vi "ChangeGraphRef.vi"(7 "NewGraphIndex":i32, 8 "error in (no error)":errorcluster caption="entrée d'erreur (pas d'erreur)", 9 "CurveIndex":i32, 11 "Interface en entrée":refnum<class "Interface.lvclass"> caption="DNL_LabVIEW Object in") -> (0 "error out":errorcluster caption="sortie d'erreur", 2 "OldGraphIndex":i32, 3 "Interface en sortie":refnum<class "Interface.lvclass"> caption="DNL_LabVIEW Object out")   [LabVIEW 2010, in "Interface.lvclass"]
uses:
  Interface.lvclass
  Interface.lvclass/Interface.ctl
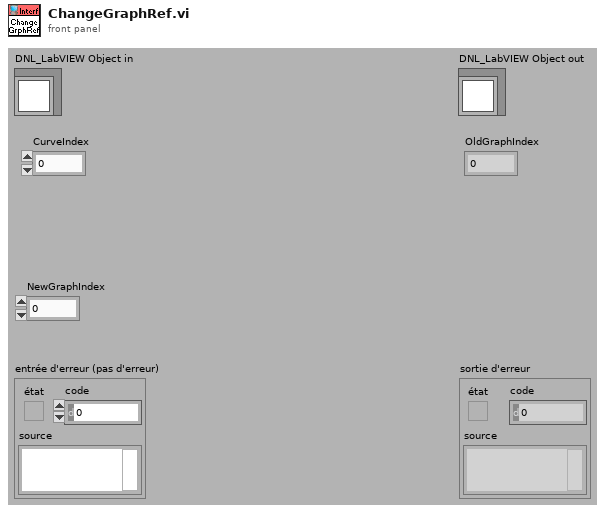
[diagram p1: front panel]
types:
  T1 = typedef "Interface.lvclass/CurveSetup.ctl" = cluster{"CurveName":string, "YParam":string, "XParam":string, "ZParam ":string, "GroupName":string, "LinWdth":u8, "PntCol":u32, "LinCol":u32, "LablFor":u8, "XScale":u32, "YScale":u32, "Interpol":u8, "DisplayName":string, "FillType":i16, "LineStyle":u8, "PntStyle":u8, "BarTyp":u8, "GraphIndex":i32, "Visible":bool, "XScaleName":string, "YScaleName":string, "XYGraph_Ref":refnum<vi>}
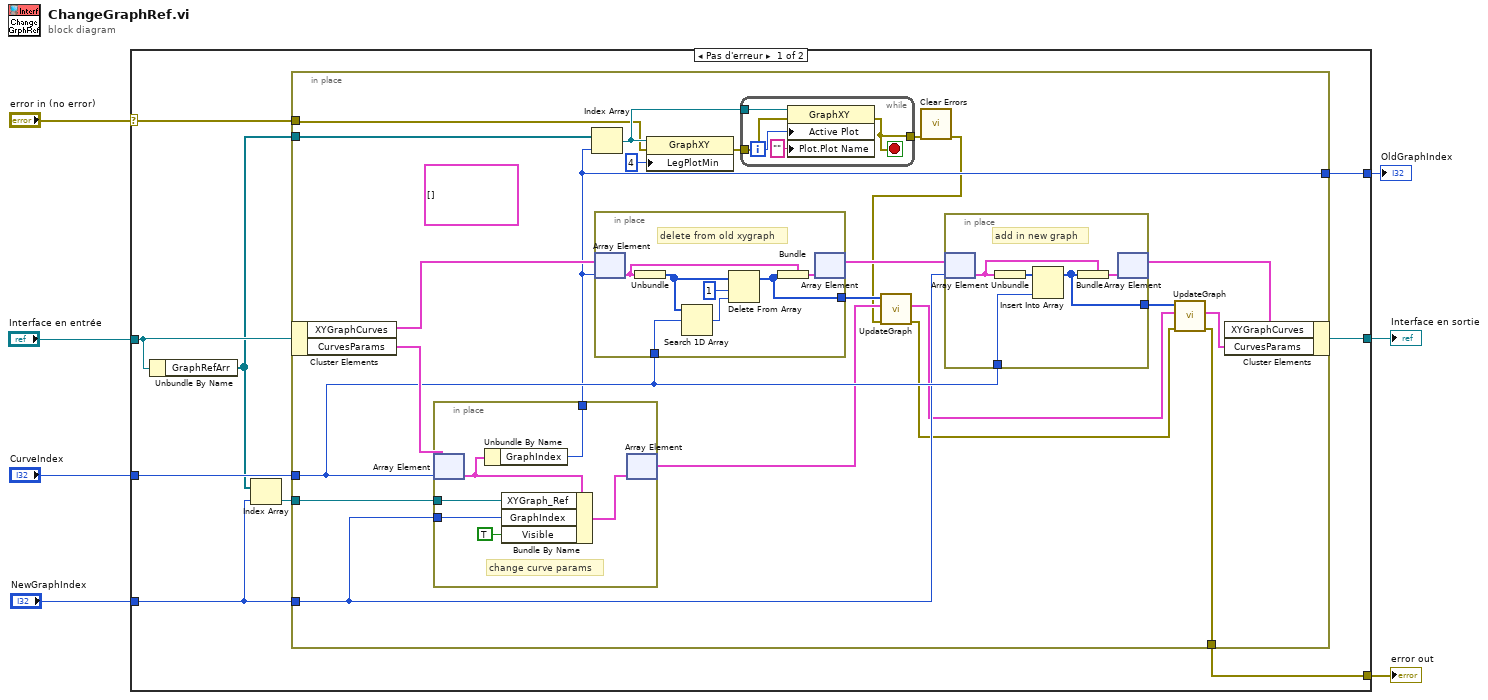
[diagram p0: block diagram]
diagram:
  n1 = case shown="Pas d'erreur" "error in (no error)" {
    selector: "error in (no error)" -> [w15 w63]
    tunnel: [w13 w63] -> w6
    tunnel: [w14 w62] -> w4
    tunnel: "Interface en entrée" -> [w12 w62]
    tunnel: "CurveIndex" -> [w16 _]
    tunnel: "NewGraphIndex" -> [w10 _]
    tunnel: [w9 _] -> w1
    frame No Error {
      n2 = Unbundle By Name(w12) -> ("GraphRefArr"=w8:refnum<vi>[])
      n3 = Index Array(array=w8, index=w10) -> (element=w11:refnum<vi>)
      n4 = in-place {
        in-place-border: w16 -> [w36]
        in-place-border: w11 -> [w37]
        in-place-border: w10 -> [w32]
        in-place-border: w15 -> [w22]
        in-place-border: [w28] -> w13
        in-place-border: [w25] -> w9
        in-place-border: w8 -> [w26]
        (unwired) cluster{dbl[], dbl[]}[] []
        n5 = in-place-cluster #1(w12) -> ("XYGraphCurves"=w35:cluster{"Tableau":i32[]}[], "CurvesParams"=w38:T1[])
        n6 = in-place {
          in-place-border: w37 -> [w60]
          in-place-border: [w58] -> w25
          in-place-border: w32 -> [w57]
          # "change curve params"
          n7 = in-place-array #2(w38, w36) -> (w59:T1)
          n8 = Unbundle By Name(w59) -> ("GraphIndex"=w58:i32)
          n9 = Bundle By Name(cluster=w59, "XYGraph_Ref"=w60, "GraphIndex"=w57, "Visible"=TRUE) -> (w61:T1)
          n10 = in-place-array #2(w61) -> (w29:T1[])  [unwired: 1 out]
        }
        n11 = Index Array(array=w26, index=w25) -> (element=w23:refnum<vi>)
        n12 = in-place {
          in-place-border: w36 -> [w54]
          in-place-border: [w49] -> w31
          # "delete from old xygraph"
          n13 = in-place-array #3(w35, w25) -> (w51:cluster{"Tableau":i32[]})
          n14 = Unbundle(w51) -> ("Tableau"=w52:i32[])
          n15 = Search 1D Array(1D array=w52, element=w54) -> (index of element=w53:i32)  [unwired: 1 in]
          n16 = Delete From Array(array=w52, length=1 ("longueur"), index=w53) -> (array with subset deleted=w49:i32[])  [unwired: 1 out]
          n17 = Bundle(cluster=w51, "Tableau"=w49) -> (w50:cluster{"Tableau":i32[]})
          n18 = in-place-array #3(w50) -> (w34:cluster{"Tableau":i32[]}[])  [unwired: 1 out]
        }
        n19 = property class="GraphXY"(reference=w23, error in=w22, "LegPlotMin"=u32 4 ("Légende : minimum de tracés")) -> (error out=w20:errorcluster)  [unwired: 1 out]
        n20 = while {
          tunnel: w23 -> [w43]
          tunnel: w20 -> [w41]
          tunnel: [w39] -> w19
          i -> [w40]
          stop <- w39 stop-if-true
          n21 = property class="GraphXY"(reference=w43, error in=w41, "Active Plot"=w40, "Plot.Plot Name"="" ("Tracé.Nom du tracé")) -> (error out=w39:errorcluster)  [unwired: 1 out]
        }
        n22 = call <vilib>:"Clear Errors.vi"("error in (no error)"=w19) -> ("error out"=w21:errorcluster)  [unwired: 6 in]
        n23 = call "UpdateGraph.vi"("error in (no error)"=w21, "CurvesParams"=w29, "CurveIndexArr"=w31) -> ("error out"=w27:errorcluster, "CurvesParamsOut"=w18:T1[])  [unwired: 7 in]
        n24 = in-place {
          in-place-border: w36 -> [w47]
          in-place-border: [w44] -> w30
          # "add in new graph"
          n25 = in-place-array #4(w34, w32) -> (w46:cluster{"Tableau":i32[]})
          n26 = Unbundle(w46) -> ("Tableau"=w48:i32[])
          n27 = Insert Into Array(array=w48, new element=w47) -> (w44:i32[])  [unwired: 1 in]
          n28 = Bundle(cluster=w46, "Tableau"=w44) -> (w45:cluster{"Tableau":i32[]})
          n29 = in-place-array #4(w45) -> (w33:cluster{"Tableau":i32[]}[])  [unwired: 1 out]
        }
        n30 = call "UpdateGraph.vi"("error in (no error)"=w27, "CurvesParams"=w18, "CurveIndexArr"=w30) -> ("error out"=w28:errorcluster, "CurvesParamsOut"=w17:T1[])  [unwired: 7 in]
        n31 = in-place-cluster #1("XYGraphCurves"=w33, "CurvesParams"=w17) -> (w14:refnum<class "Interface.lvclass">)
      }
    }
    frame Error {
    }
  }
  "error out" <- w6
  "Interface en sortie" <- w4
  "OldGraphIndex" <- w1
